vi "Refresh Is Frame in ECU.vi"(7 "ECU Name":string, 8 "Type (Input)":T3, 9 "Frame":T1, 10 "Frames":T1[](array[typedef]), 11 "ECUs":T4[](array[typedef])) -> (3 "Found?":bool)   [LabVIEW 2020, in "Communication Bus Template System Explorer.lvlib" / "Implementation.lvlib"]
uses:
  Implementation.lvlib
  Types/ECU.ctl
  <vilib>/NI VeriStand/Custom Device API/Custom Device Channel Type.ctl
  Types/Frame.ctl
  Types/Signal.ctl
  <vilib>/NI VeriStand/Custom Device API/Custom Device API.lvlib
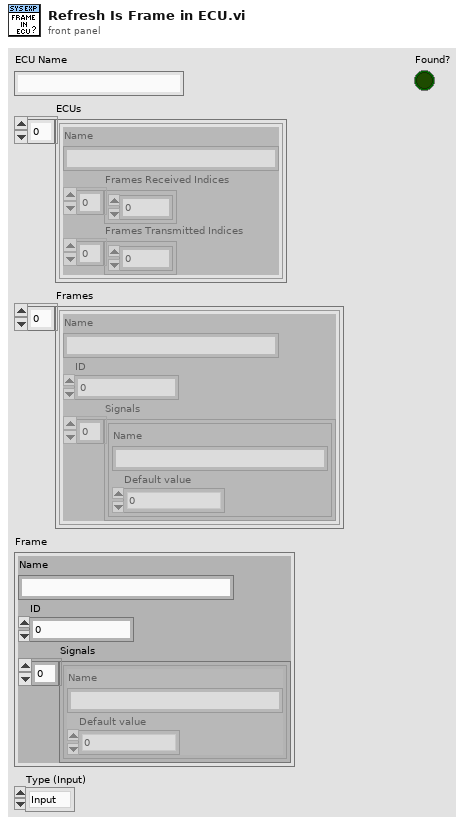
[diagram p1: front panel]
types:
  T1 = typedef "Communication Bus Template System Explorer.lvlib/Implementation.lvlib/Frame.ctl" = cluster{"Name":string, "ID":u32, "Signals":T2[]}
  T2 = typedef "Communication Bus Template System Explorer.lvlib/Implementation.lvlib/Signal.ctl" = cluster{"Name":string, "Default value":dbl}
  T3 = typedef "Custom Device API.lvlib/Custom Device Channel Type.ctl" = enum16{"Input", "Output"}
  T4 = typedef "Communication Bus Template System Explorer.lvlib/Implementation.lvlib/ECU.ctl" = cluster{"Name":string, "Frames Received Indices":u32[], "Frames Transmitted Indices":u32[]}
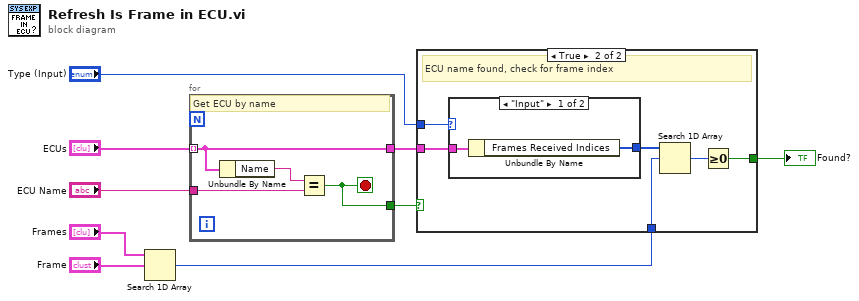
[diagram p0: block diagram]
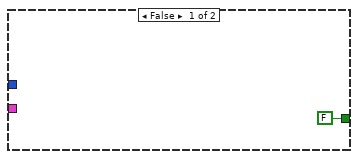
[diagram p2: hidden frame]
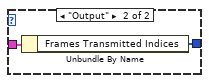
[diagram p3: hidden frame]
diagram:
  n1 = Search 1D Array(1D array="Frames", element="Frame") -> (index of element=w3:i32)  [unwired: 1 in]
  n2 = for {
    tunnel: "ECUs" -> [w11] mode=indexing
    tunnel: "ECU Name" -> [w12]
    tunnel: [w11] -> w4
    tunnel: [w10] -> w2
    stop <- w10 stop-if-true
    # "Get ECU by name"
    n3 = Unbundle By Name(w11) -> ("Name"=w13:string)
    n4 = Equal?(x=w13, y=w12) -> (x = y?=w10:bool)
  }
  n5 = case shown="True" w2 {
    tunnel: "Type (Input)" -> [_ w18]
    tunnel: w4 -> [_ w17]
    tunnel: w3 -> [_ w16]
    tunnel: [FALSE w15] -> w1
    frame False {
    }
    frame True {
      # "ECU name found, check for frame index"
      n6 = case shown="\"Input\"" w18 {
        tunnel: w17 -> [w22 w24]
        tunnel: [w21 w23] -> w19
        frame "Input" {
          n7 = Unbundle By Name(w22) -> ("Frames Received Indices"=w21:u32[])
        }
        frame "Output" {
          n8 = Unbundle By Name(w24) -> ("Frames Transmitted Indices"=w23:u32[])
        }
      }
      n9 = Search 1D Array(1D array=w19, element=w16) -> (index of element=w20:i32)  [unwired: 1 in]
      n10 = Greater Or Equal To 0?(x=w20) -> (x >= 0?=w15:bool)
    }
  }
  "Found?" <- w1
